vi "Get Routing.vi"(2 "shared":refnum<class "niUSRP Rx Core v1 FPGA.lvclass">=refnum) -> (4 "routing":refnum<class "niVST Routing (Base) v1 FPGA.lvclass">)   [LabVIEW 2023]
doc: "this VI is an accessor for the Routing class handle."
uses:
  <instrlib>/niUSRP/Reference FPGA/Rx Core/niUSRP Rx Core v1 FPGA.lvclass
  <instrlib>/niVST/Reference FPGA/FPGA/Routing/v1/Base/niVST Routing (Base) v1 FPGA.lvclass
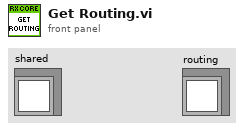
[diagram p1: front panel]
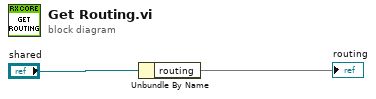
[diagram p0: block diagram]
diagram:
  n1 = Unbundle By Name("shared") -> ("routing"=→"routing")
